vi "loop_display.vi"(8 "error in":errorcluster, 9 "timing source":string="1 kHz", 11 "reference cluster":T1) -> ()   [LabVIEW 2016]
uses:
  Type Definitions/reference_cluster.ctl
  Type Definitions/vars_settings.ctl
  Type Definitions/stim_type.ctl
  Type Definitions/vars_runtime.ctl
  Type Definitions/data.ctl
  Type Definitions/notifier_elements_GUI.ctl
  Type Definitions/notifier_elements_DAQ.ctl
  Type Definitions/notifier_elements_write.ctl
  Type Definitions/control_references.ctl
  <vilib>/Platform/TimedLoop/XDataNode/timing_clust.ctl
  <vilib>/Platform/TimedLoop/XDataNode/nitl_modes.ctl
  <vilib>/Platform/TimedLoop/XDataNode/wakeup.ctl
  <vilib>/Platform/TimedLoop/XDataNode/XDataNode.xnode
  <vilib>/Platform/TimedLoop/XDataNode/XDNodeRunTimeDep.lvlib
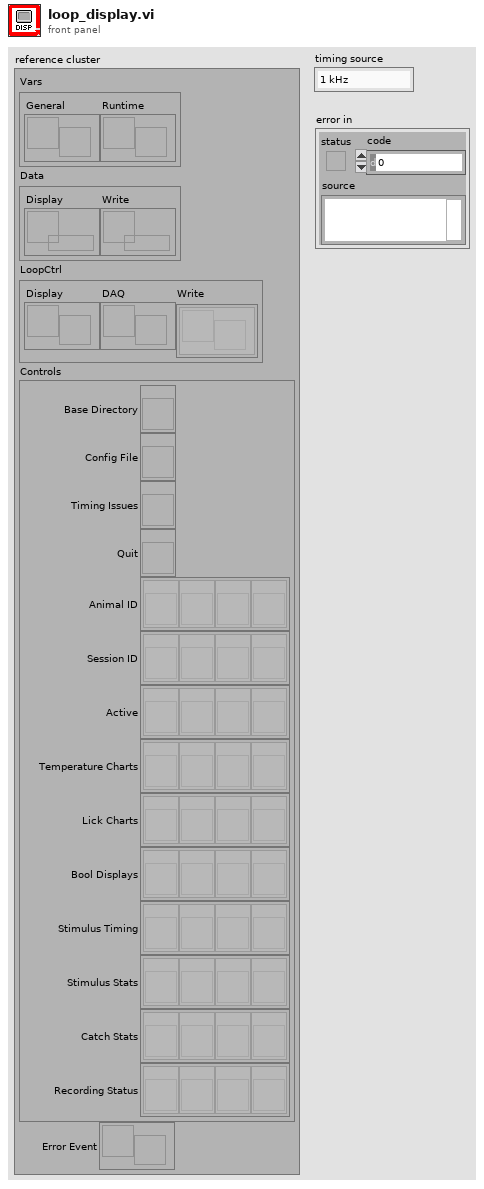
[diagram p1: front panel]
types:
  T1 = typedef "reference_cluster.ctl" = cluster{"Vars":cluster{"General":refnum<notifier>, "Runtime":refnum<notifier>}, "Data":cluster{"Display":refnum<queue>, "Write":refnum<queue>}, "LoopCtrl":cluster{"Display":refnum<notifier>, "DAQ":refnum<notifier>, "Write":refnum<notifier>[]}, "Controls":T2, "Error Event":refnum<user-event>}
  T2 = typedef "control_references.ctl" = cluster{"Base Directory":refnum<vi>, "Config File":refnum<vi>, "Timing Issues":refnum<vi>, "Quit":refnum<vi>, "Animal ID":refnum<vi>[], "Session ID":refnum<vi>[], "Active":refnum<vi>[], "Temperature Charts":refnum<vi>[], "Lick Charts":refnum<vi>[], "Bool Displays":refnum<vi>[], "Stimulus Timing":refnum<vi>[], "Stimulus Stats":refnum<vi>[], "Catch Stats":refnum<vi>[], "Recording Status":refnum<vi>[]}
  T3 = typedef "XDNodeRunTimeDep.lvlib/timing_clust.ctl" = cluster{"Expected End [f-1]":u64, "Actual End [f-1]":u64, "Finished Late? [f-1]":bool, "Expected End [i-1]":u64, "Actual End [i-1]":u64, "Finished Late? [i-1]":bool, "Expected Start [i]":u64, "Actual Start [i]":u64, "Expected Start [f]":u64, "Actual Start [f]":u64, "Source Name":string, "Structure Name":string, "Period":i64, "Deadline":i64, "Offset":i64, "Start":i64, "Priority":i32, "Timeout":i32, "Mode":T4, "Wakeup Reason":T5, "Error":errorcluster, "Source Type":string, "Secondary Source Type":string, "Global End Time":u64, "Global Start Time":u64, "Frame Duration":u64, "Iteration Duration":u64, "Assigned CPU":i32, "I/O Scan Engine Mode":u32}
  T4 = typedef "XDNodeRunTimeDep.lvlib/nitl_modes.ctl" = enum32{"No Change", "Process missed periods, maintain original phase", "Discard missed periods, maintain original phase", "Process missed periods, ignore original phase", "Discard missed periods, ignore original phase"}
  T5 = typedef "XDNodeRunTimeDep.lvlib/wakeup.ctl" = enum32{"Normal", "Aborted", "Asynchronous wakeup", "Timing source error", "Timed loop error", "Timeout"}
  T6 = typedef "notifier_elements_GUI.ctl" = enum16{"Initialize GUI", "Pause", "Live Update", "Stat Update", "Quit"}
  T7 = typedef "vars_settings.ctl" = cluster{"base directory":path, "data directory":path, "active":bool, "running":bool, "pairing":bool, "clean tubes":bool, "animal ID":u16, "session ID":u16, "base temp":dbl, "d wait min":u16, "d wait max":u16, "d timeout":u16, "d reward":u16, "idx stim":u16, "timeout win":u16, "lick win":i32[], "stim type":T8[], "stim dur":u16[], "stim amp":dbl[], "stim freq":u16[], "stim ramp":u16[], "stim catch":u8[], "square dur":u8[], "square delay":u8[], "square freq":u8[], "square dc":u8[], "stim shape":dbl[][], "square shape":bool[][]}
  T8 = typedef "stim_type.ctl" = enum16{"pulse", "vibration", "square", "sine"}
  T9 = typedef "data.ctl" = cluster{"time":u32, "finished late":bool, "temp out":sgl[], "temp in":sgl[], "lick in":sgl[], "stim":bool[], "catch":bool[], "lick":bool[], "reward":bool[], "backlight":bool[], "freqstim":bool[]}
  T10 = cluster{"stim":bool, "catch":bool, "square":bool, "lick":bool, "reward":bool}[]
  T11 = typedef "vars_runtime.ctl" = cluster{"t wait":u16, "t stim":u16, "t square":u16, "t reward":u16, "t since onset":u16, "n stim":u16, "n hit":u16, "n miss":u16, "n catch":u16, "n reject":u16, "n false alarm":u16, "stim amp":sgl, "stim idx":i32, "next temp":sgl, "catch":bool, "stimulus":bool, "reward given":bool, "lick":bool, "next reward":bool, "backlight":bool, "square":bool, "first run?":bool, "d stim":u16, "t rel":u16, "d square":u16}
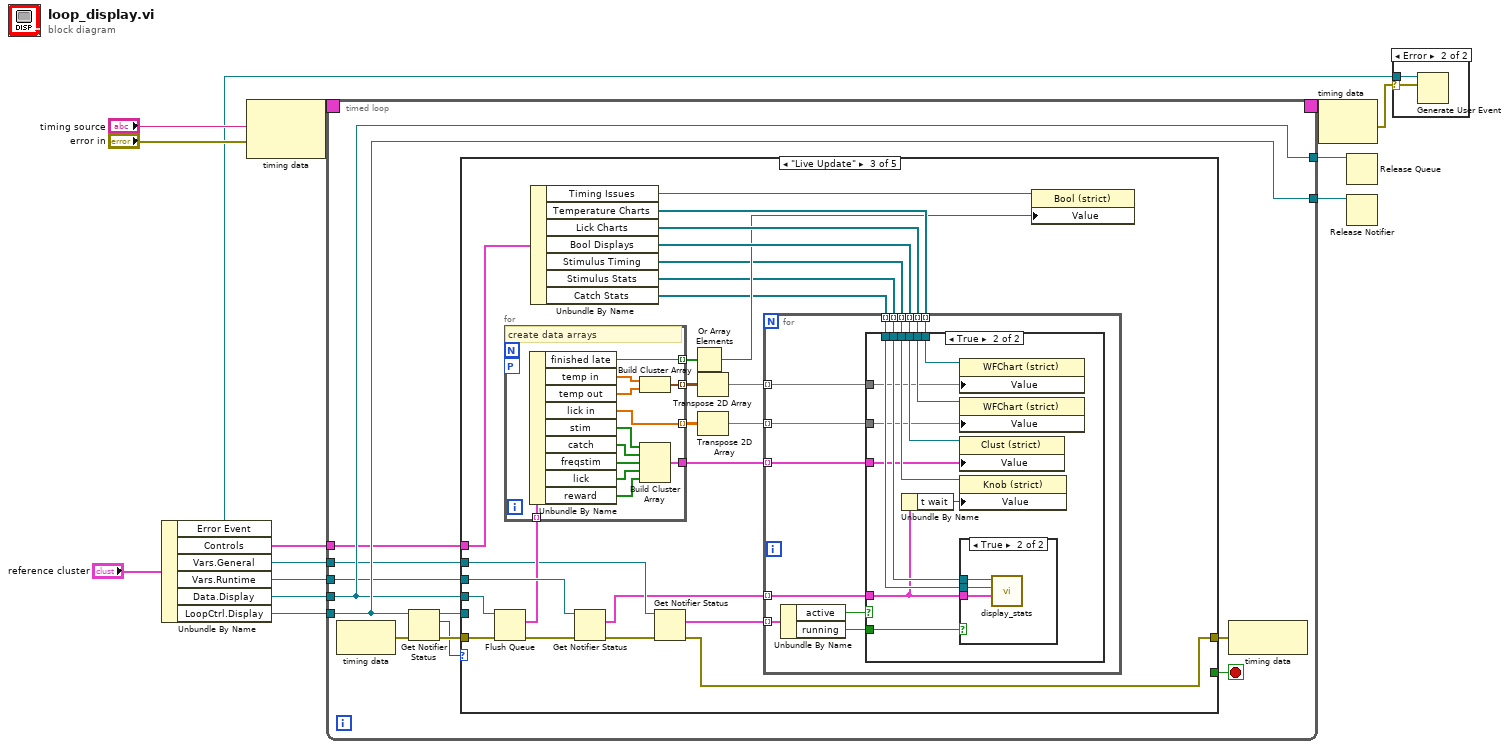
[diagram p0: block diagram]
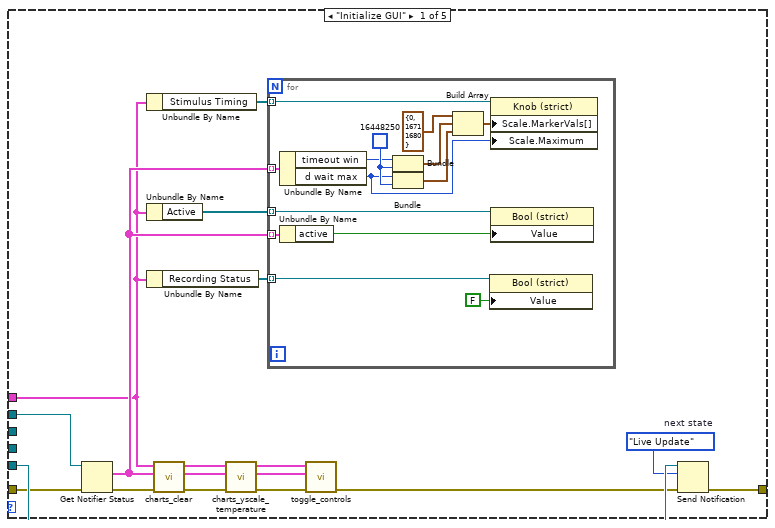
[diagram p3: hidden frame]
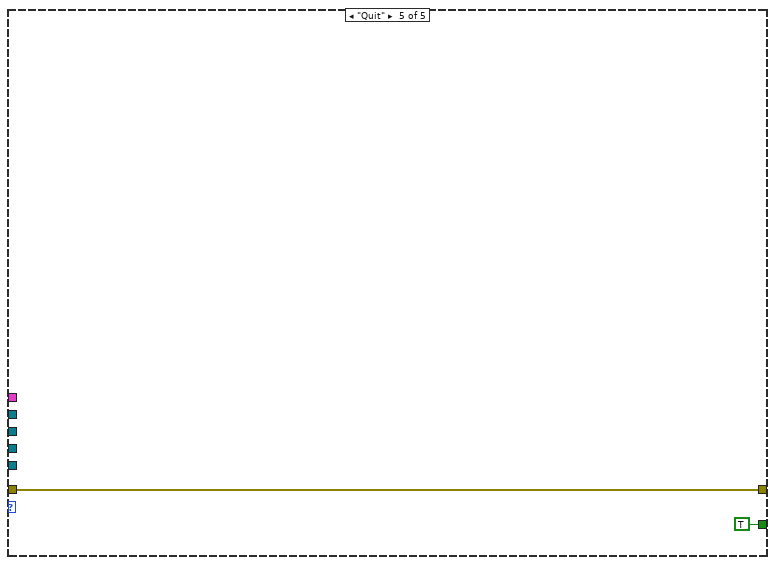
[diagram p8: hidden frame]
diagram:
  n1 = Unbundle By Name("reference cluster") -> ("Error Event"=w2:refnum<user-event>, "Controls"=w6:T2, "Vars.General"=w7:refnum<notifier>, "Vars.Runtime"=w4:refnum<notifier>, "Data.Display"=w3:refnum<queue>, "LoopCtrl.Display"=w5:refnum<notifier>)
  n2 = node-c288("timing source", "error in") -> (w14:T3)
  n3 = timed-loop "Display" {
    timing: w14 -> [_]
    timing-out: [_] -> w13
    tunnel: w7 -> [w23]
    tunnel: w6 -> [w22]
    tunnel: [w25] -> w10
    tunnel: [w24] -> w9
    tunnel: w5 -> [w25]
    tunnel: w4 -> [w15]
    tunnel: w3 -> [w24]
    stop <- w21 stop-if-true
    n4 = node-c288() -> (w20:errorcluster)  [unwired: 1 in]
    n5 = Get Notifier Status(notifier=w25, error in (no error)=w20) -> (notifier out=w19:refnum<notifier>, current notification=w17:T6, error out=w18:errorcluster)  [unwired: 2 out]
    n6 = case shown="\"Live Update\"" w17 {
      tunnel: w23 -> [w38 _ w67 _ _]
      tunnel: [w42 w58 w68 w124 w125] -> w16
      tunnel: w22 -> [w27 _ w64 _ _]
      tunnel: [_ _ _ _ TRUE] -> w21
      tunnel: w19 -> [w43 _ _ _ _]
      tunnel: w18 -> [w39 w58 w83 w124 w125]
      tunnel: w15 -> [_ _ w82 _ _]
      tunnel: w24 -> [_ _ w59 _ _]
      frame "Initialize GUI" {
        w41 = notifier_elements_GUI."Live Update"  # next state
        n7 = Get Notifier Status(notifier=w38, error in (no error)=w39) -> (current notification=w28:T7[], error out=w37:errorcluster)  [unwired: 3 out]
        n8 = Unbundle By Name(w27) -> ("Stimulus Timing"=w29:refnum<vi>[])
        n9 = Unbundle By Name(w27) -> ("Active"=w30:refnum<vi>[])
        n10 = Unbundle By Name(w27) -> ("Recording Status"=w26:refnum<vi>[])
        n11 = call "charts_clear.vi"("error in"=w37, "vars general"=w28, "control cluster"=w27) -> ("error out"=w40:errorcluster, "vars general"=w35:T7[], "control cluster"=w36:T2)  [unwired: 6 in]
        n12 = call "charts_yscale_temperature.vi"("error in"=w40, "vars general"=w35, "control cluster"=w36) -> ("error out"=w34:errorcluster, "vars general"=w33:T7[], "control cluster"=w32:T2)  [unwired: 6 in]
        n13 = for {
          tunnel: w30 -> [w57] mode=indexing
          tunnel: w28 -> [w56] mode=indexing
          tunnel: w29 -> [w54] mode=indexing
          tunnel: w28 -> [w53] mode=indexing
          tunnel: w26 -> [w44] mode=indexing
          w49 = u32 16448250
          n14 = Unbundle By Name(w53) -> ("timeout win"=w48:u16, "d wait max"=w46:u16)
          n15 = Unbundle By Name(w56) -> ("active"=w55:bool)
          n16 = Bundle("timeout win"=w48, w49) -> (w50:cluster{"timeout win":u16, u32})  [unwired: 1 in]
          n17 = Bundle("d wait max"=w46, w49) -> (w51:cluster{"d wait max":u16, u32})  [unwired: 1 in]
          n18 = Build Array(cluster{u16, u32} {0, 16711680}, w50, w51) -> (w52:cluster{"d wait max":u16, u32}[])
          n19 = property class="Bool (strict)"(reference=w44, "Value"=FALSE) -> ()  [unwired: 1 in, 2 out]
          n20 = property class="Knob (strict)"(reference=w54, "Scale.MarkerVals[]"=w52, "Scale.Maximum"=w46) -> ()  [unwired: 1 in, 2 out]
          n21 = property class="Bool (strict)"(reference=w57, "Value"=w55) -> ()  [unwired: 1 in, 2 out]
        }
        n22 = call "toggle_controls.vi"("error in"=w34, "vars general in"=w33, "control cluster in"=w32) -> ("error out"=w31:errorcluster)  [unwired: 5 in, 3 out]
        n23 = Send Notification(notification=w41, notifier=w43, error in (no error)=w31) -> (error out=w42:errorcluster)  [unwired: 1 out]
      }
      frame "Pause" {
      }
      frame "Live Update" {
        n24 = Flush Queue(queue=w59, error in (no error)=w83) -> (remaining elements=w81:T9[], error out=w72:errorcluster)  [unwired: 1 out]
        n25 = for {
          tunnel: w81 -> [w123] mode=indexing
          tunnel: [w118] -> w80 mode=indexing
          tunnel: [w122] -> w78 mode=indexing
          tunnel: [w121] -> w75 mode=indexing
          workers-P: _ -> [_]
          tunnel: [w117] -> w61
          # "create data arrays"
          n26 = Unbundle By Name(w123) -> ("finished late"=w121:bool, "temp in"=w120:sgl[], "temp out"=w119:sgl[], "lick in"=w122:sgl[], "stim"=w113:bool[], "catch"=w114:bool[], "freqstim"=w115:bool[], "lick"=w116:bool[], "reward"=w112:bool[])
          n27 = Build Cluster Array(w120, w119) -> (w118:cluster{"temp in":sgl, "temp out":sgl}[])
          n28 = Build Cluster Array(w113, w114, w115, w116, w112) -> (w117:T10)
        }
        n29 = Unbundle By Name ("get indicator references")(w64) -> ("Timing Issues"=w71:refnum<vi>, "Temperature Charts"=w79:refnum<vi>[], "Lick Charts"=w77:refnum<vi>[], "Bool Displays"=w76:refnum<vi>[], "Stimulus Timing"=w73:refnum<vi>[], "Stimulus Stats"=w63:refnum<vi>[], "Catch Stats"=w62:refnum<vi>[])
        n30 = Get Notifier Status(notifier=w82, error in (no error)=w72) -> (current notification=w65:T11[], error out=w69:errorcluster)  [unwired: 3 out]
        n31 = Get Notifier Status(notifier=w67, error in (no error)=w69) -> (current notification=w66:T7[], error out=w68:errorcluster)  [unwired: 3 out]
        n32 = Or Array Elements(Boolean array=w75) -> (logical OR=w74:bool)
        n33 = Transpose 2D Array(2D array=w80) -> (transposed array=w70:cluster{"temp in":sgl, "temp out":sgl}[][])
        n34 = Transpose 2D Array(2D array=w78) -> (transposed array=w60:sgl[][])
        n35 = for {
          tunnel: w70 -> [w95] mode=indexing
          tunnel: w79 -> [w96] mode=indexing
          tunnel: w60 -> [w94] mode=indexing
          tunnel: w77 -> [w93] mode=indexing
          tunnel: w76 -> [w92] mode=indexing
          tunnel: w73 -> [w91] mode=indexing
          tunnel: w65 -> [w87] mode=indexing
          tunnel: w61 -> [w90] mode=indexing
          tunnel: w66 -> [w89] mode=indexing
          tunnel: w63 -> [w84] mode=indexing
          tunnel: w62 -> [w85] mode=indexing
          # "write data to indicators"
          n36 = Unbundle By Name(w89) -> ("active"=w88:bool, "running"=w86:bool)
          n37 = case shown="True" w88 {
            tunnel: w96 -> [_ w103]
            tunnel: w95 -> [_ w102]
            tunnel: w94 -> [_ w101]
            tunnel: w93 -> [_ w108]
            tunnel: w92 -> [_ w107]
            tunnel: w91 -> [_ w106]
            tunnel: w90 -> [_ w97]
            tunnel: w87 -> [_ w98]
            tunnel: w86 -> [_ w99]
            tunnel: w85 -> [_ w105]
            tunnel: w84 -> [_ w104]
            frame False {
              # "setup is disabled"
            }
            frame True {
              # "setup is active"
              n38 = Unbundle By Name(w98) -> ("t wait"=w100:u16)
              n39 = property class="WFChart (strict)"(reference=w103, "Value"=w102) -> ()  [unwired: 1 in, 2 out]
              n40 = property class="WFChart (strict)"(reference=w108, "Value"=w101) -> ()  [unwired: 1 in, 2 out]
              n41 = property class="Clust (strict)"(reference=w107, "Value"=w97) -> ()  [unwired: 1 in, 2 out]
              n42 = property class="Knob (strict)"(reference=w106, "Value"=w100) -> ()  [unwired: 1 in, 2 out]
              n43 = case shown="True" w99 {
                tunnel: w98 -> [_ w109]
                tunnel: w105 -> [_ w110]
                tunnel: w104 -> [_ w111]
                frame False {
                  # "no new stats are available"
                }
                frame True {
                  # "new stats are available"
                  n44 = call "display_stats.vi"("Variables"=w109, "catch stats"=w110, "stim stats"=w111) -> ()  [unwired: 8 in, 1 out]
                }
              }
            }
          }
        }
        n45 = property on="Property Node" class="Bool (strict)"(reference=w71, "Value"=w74) -> ()  [unwired: 1 in, 2 out]
      }
      frame "Stat Update" {
      }
      frame "Quit" {
      }
    }
    n46 = node-c288(w16) -> ()  [unwired: 1 out]
  }
  n47 = node-c288(w13) -> (w1:errorcluster)
  n48 = Release Queue(queue=w9) -> ()  [unwired: 2 in, 3 out]
  n49 = Release Notifier(notifier=w10) -> ()  [unwired: 2 in, 3 out]
  n50 = case shown="Error" w1 {
    selector: w1 -> [_ w132]
    tunnel: w2 -> [_ w133]
    frame No Error {
    }
    frame Error {
      n51 = Generate User Event(user event=w133, event data cluster=w132) -> ()  [unwired: 2 in, 2 out]
    }
  }
